vi "destroy.vi"(8 "error in":errorcluster, 11 "MultiPart Upload":refnum<class "Multipart Upload.lvclass">) -> (0 "error out":errorcluster)   [LabVIEW 2020, in "Multipart Upload.lvclass"]
uses:
  Multipart Upload.lvclass
  Multipart Upload.lvclass/Multipart Upload.ctl
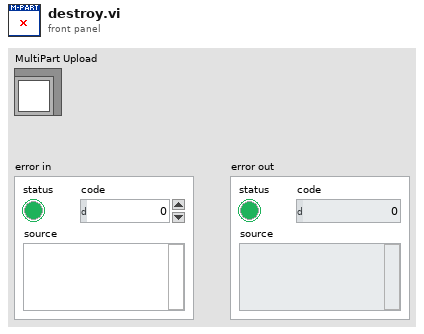
[diagram p1: front panel]
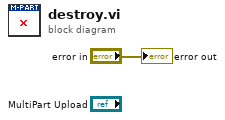
[diagram p0: block diagram]
diagram:
  "error out" <- "error in"
